vi "AbsLimit (SubVI).vi"(10 "in":i32, 11 "Abslimt":i32) -> (3 "Numeric out":i32)   [LabVIEW 2021]
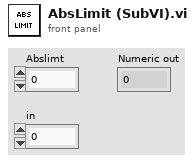
[diagram p1: front panel]
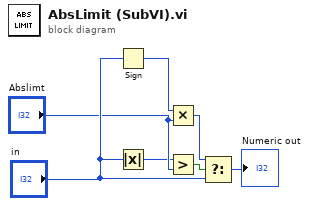
[diagram p0: block diagram]
diagram:
  n1 = Sign(1:"in") -> (0:w5:i32)
  n2 = Absolute Value(x="in") -> (abs(x)=w1:i32)
  n3 = Multiply(x=w5, y="Abslimt") -> (x*y=w4:i32)
  n4 = Greater?(x=w1, y="Abslimt") -> (0:w2:bool)
  n5 = Select(t=w4, s=w2, f="in") -> (s? t:f=→"Numeric out":i32)
